vi "Winch Oper.vi"   [LabVIEW 2016]
uses:
  Robot Global Data.vi
types:
  T1 = typedef "WPI_DriverStationRobotMode2.ctl" = enum16{"Autonomous Disabled", "Autonomous Enabled", "Teleop Disabled", "Teleop Enabled", "Disconnected", "Finish", "Test Disabled", "Test Enabled", "Emergency Stopped"}
  T2 = typedef "WPI_MotorControlDeviceRef.ctl" = cluster{"DeviceStatus":errorcluster, "Type":T3, "PWM":cluster{"PWM Channel":T4, "DeadBand":T5}, "CAN":cluster{"Device Number":u8, "SetOutput VI Ref":variant, "GetOutput VI Ref":variant, "Enable VI Ref":variant, "Disable VI Ref":variant, "Data":variant}, "Invert":bool}
  T3 = typedef "WPI_MotorControlType.ctl" = enum16{"PWM", "CAN"}
  T4 = typedef "FPGA_DIOPWMChannel.ctl" = enum8{"PWM 0", "PWM 1", "PWM 2", "PWM 3", "PWM 4", "PWM 5", "PWM 6", "PWM 7", "PWM 8", "PWM 9", "PWM MXP 0", "PWM MXP 1", "PWM MXP 2", "PWM MXP 3", "PWM MXP 4", "PWM MXP 5", "PWM MXP 6", "PWM MXP 7", "PWM MXP 8", "PWM MXP 9", "Invalid"}
  T5 = typedef "WPI_PWMDeadband.ctl" = cluster{"Name":string, "maxPositivePwm":i32, "minPositivePwm":i32, "centerPwm":i32, "maxNegativePwm":i32, "minNegativePwm":i32, "angularRange":u16}
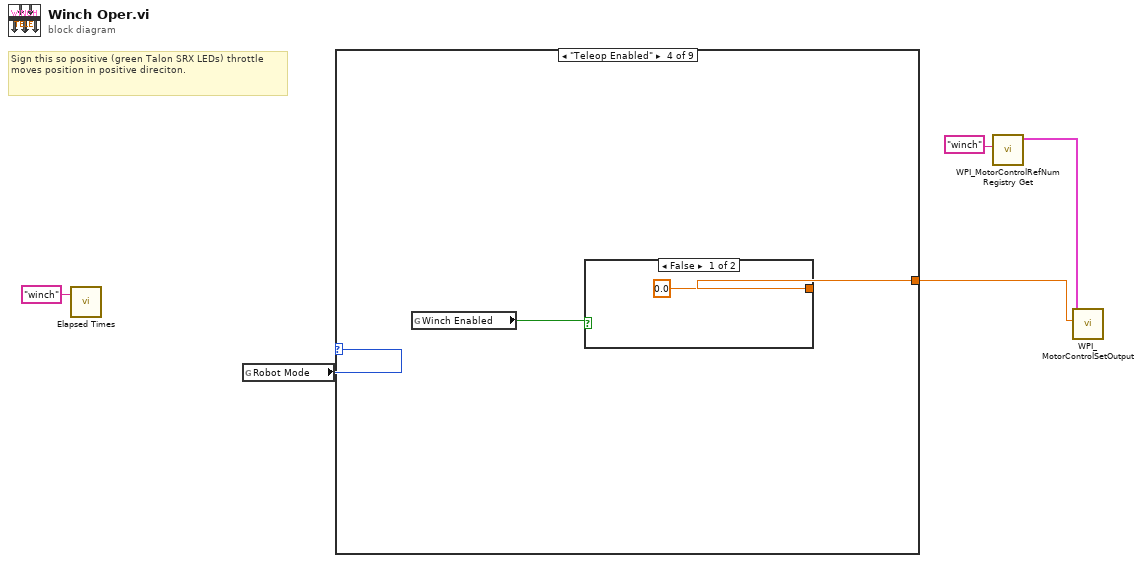
[diagram p0: block diagram]
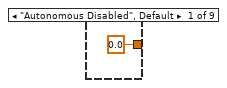
[diagram p2: hidden frame]
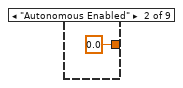
[diagram p3: hidden frame]
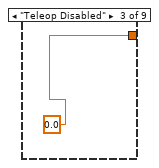
[diagram p4: hidden frame]
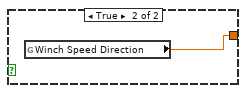
[diagram p5: hidden frame]
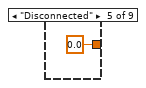
[diagram p6: hidden frame]
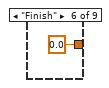
[diagram p7: hidden frame]
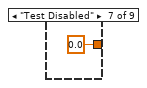
[diagram p8: hidden frame]
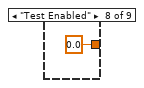
[diagram p9: hidden frame]
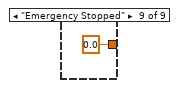
[diagram p10: hidden frame]
diagram:
  # "Sign this so positive (green Talon SRX LEDs) throttle moves position in positive direciton."
  n1 = call "Elapsed Times.vi"("Call Name"="winch") -> ()  [unwired: 2 in, 1 out]
  n2 = global read "Robot Global Data.vi" "Robot Mode"() -> (w5:T1)
  n3 = case shown="\"Teleop Enabled\"" w5 {
    tunnel: [0.0 ("upper limit") 0.0 ("upper limit") 0.0 ("upper limit") w10 0.0 ("upper limit") 0.0 ("upper limit") 0.0 ("upper limit") 0.0 ("upper limit") 0.0 ("upper limit")] -> w4
    frame "Autonomous Disabled", Default {
    }
    frame "Autonomous Enabled" {
    }
    frame "Teleop Disabled" {
    }
    frame "Teleop Enabled" {
      n4 = global read "Robot Global Data.vi" "Winch Enabled"() -> (w9:bool)
      n5 = case shown="False" w9 {
        tunnel: [0.0 ("upper limit") w12] -> w10
        frame False {
        }
        frame True {
          n6 = global read "Robot Global Data.vi" "Winch Speed Direction"() -> (w12:dbl)
        }
      }
    }
    frame "Disconnected" {
    }
    frame "Finish" {
    }
    frame "Test Disabled" {
    }
    frame "Test Enabled" {
    }
    frame "Emergency Stopped" {
    }
  }
  n7 = call <vilib>:"WPI_MotorControlRefNum Registry Get.vi"("refnum name"="winch") -> ("MotorControlDevRef"=w2:T2)  [unwired: 9 in, 1 out]
  n8 = call <vilib>:"WPI_MotorControlSetOutput.vi"("Output"=w4, "MotorControlDevRef"=w2) -> ()  [unwired: 7 in, 3 out]
